vi "Boiler.vi"() -> ()   [LabVIEW 2023]
uses:
  Controls/Boiler Controls.ctl
  Controls/Boiler Simulation Controls.ctl
  Controls/Boiler Status Indicators.ctl
  Controls/State.ctl
  Controls/DataCluster.ctl
panel:
  out "error out":errorcluster
  in  "error in (no error)":errorcluster
  in  "stop":bool
  out "Boiler Status Indicators":T1={"Status"="Lockout", "Primary Fan"=FALSE, "Natural Gas Valve"=FALSE, "Pilot"=FALSE, "Fuel Valve"=FALSE, "Forced Draft Fan"=FALSE, "Time Count"=0.0} {"Time Count" format="%.2g"}
  in  "Boiler Simulation Controls":T2 {"Flame Sensor Value (%)" min=0.0 max=100.0 scale=0.0..100.0}
  in  "Boiler Controls":T3 {"Fuel Valve Position" min=0.0 max=100.0 scale=0.0..100.0 scale format="%.2f"}
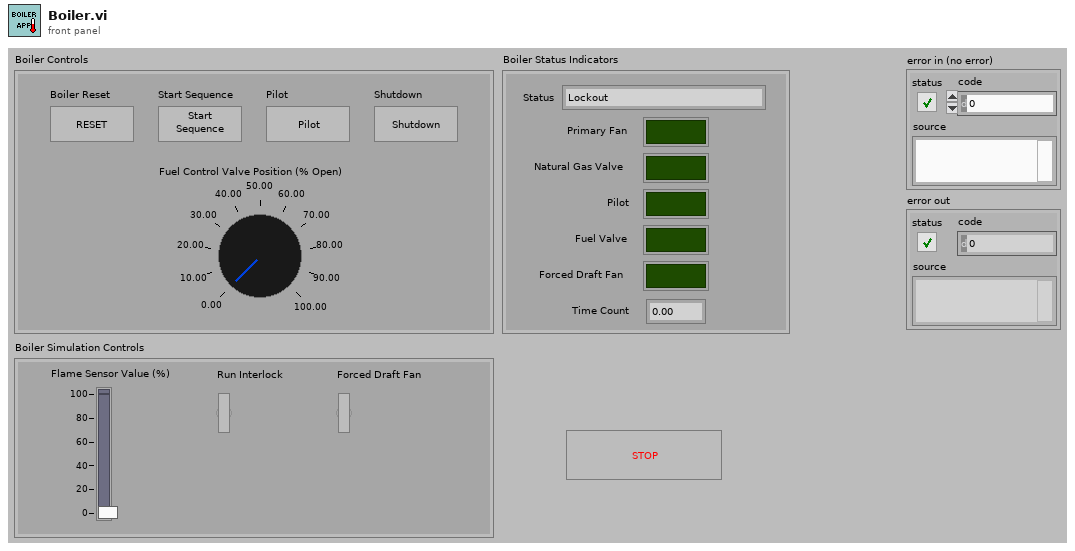
[diagram p1: front panel]
types:
  T1 = typedef "Boiler Status Indicators.ctl" = cluster{"Status":string, "Primary Fan":bool, "Natural Gas Valve":bool, "Pilot":bool, "Fuel Valve":bool, "Forced Draft Fan":bool, "Time Count":dbl}
  T2 = typedef "Boiler Simulation Controls.ctl" = cluster{"Flame Sensor Value (%)":dbl, "Run Interlock":bool, "Forced Draft Fan":bool}
  T3 = typedef "Boiler Controls.ctl" = cluster{"Boiler Reset":bool, "Start Sequence":bool, "Pilot":bool, "Shutdown":bool, "Fuel Valve Position":dbl}
  T4 = typedef "DataCluster.ctl" = cluster{"Boiler Log Path":path, "Last State":T5, "Time out":i32, "Ini Values":cluster{"Timer Count":dbl, "Flame Range Value":dbl, "Valve Position ":cluster{"Min":dbl, "Max":dbl}}, "Flame Sensor Val":dbl, "Fuel Valve Position":dbl, "Timeout Rate":i32}
  T5 = typedef "State.ctl" = enum16{"Boiler Initialized", "Boiler Ready", "Start Pre-Purge", "Pre-Purge Complete", "Pilot On", "Pilot Proved", "Force Draft Fan ON", "Boiler Running", "Start Shutdown Purge", "Shutdown Purge Complete", "Wait for Something"}
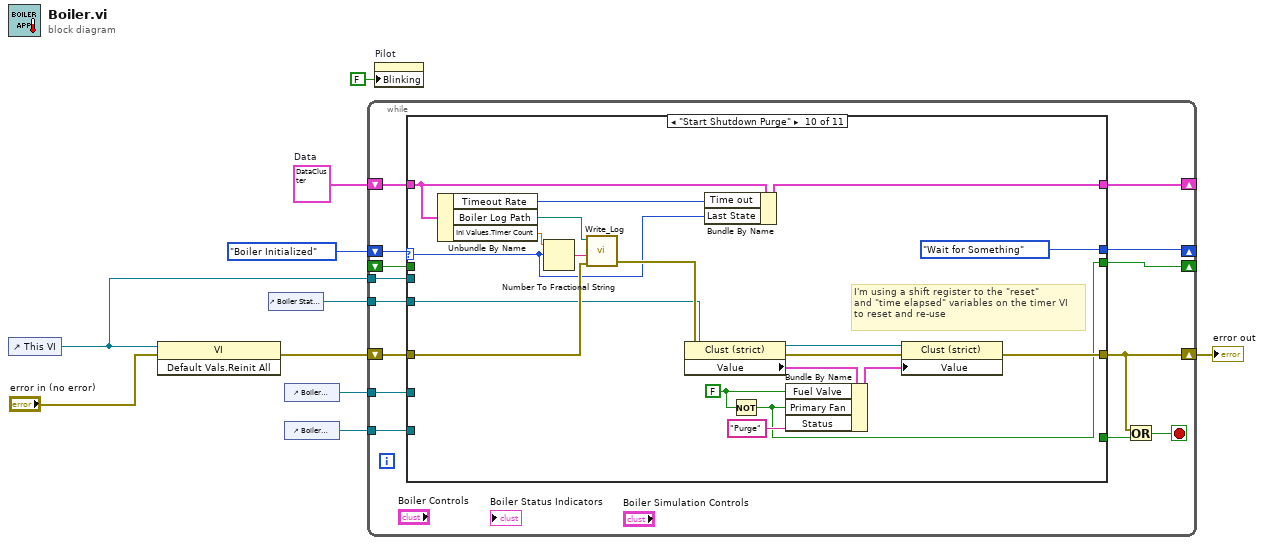
[diagram p0: block diagram]
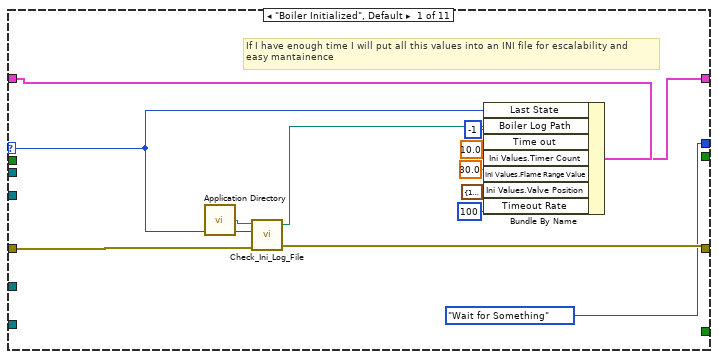
[diagram p2: hidden frame]
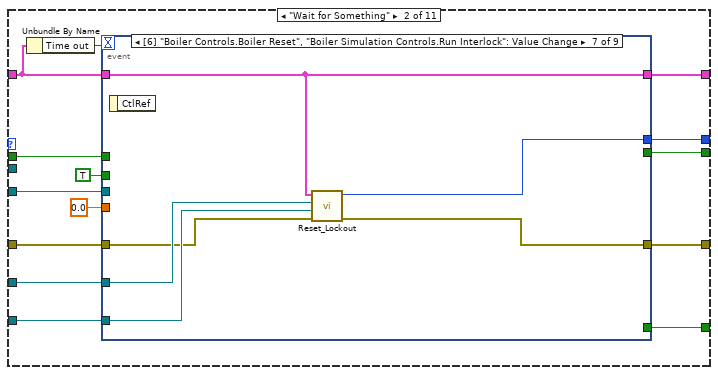
[diagram p3: hidden frame]
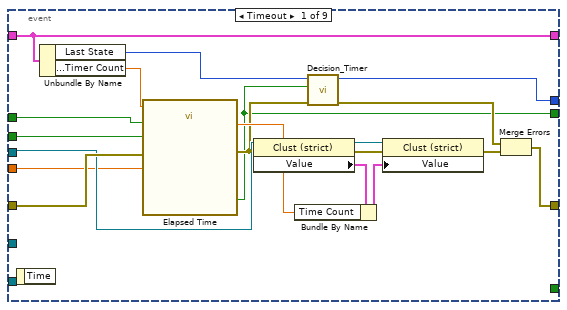
[diagram p4: hidden frame]
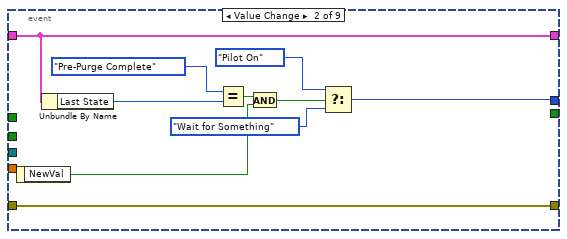
[diagram p5: hidden frame]
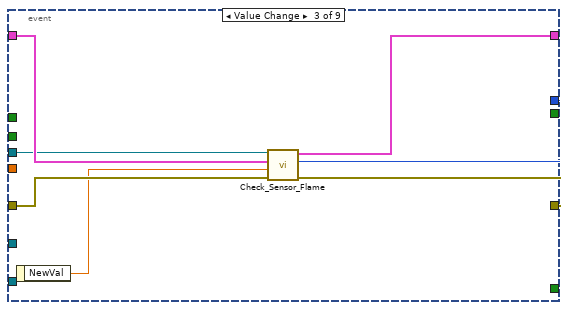
[diagram p6: hidden frame]
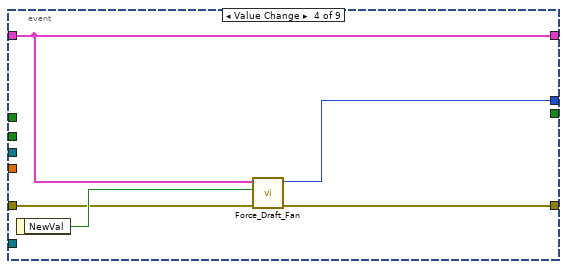
[diagram p7: hidden frame]
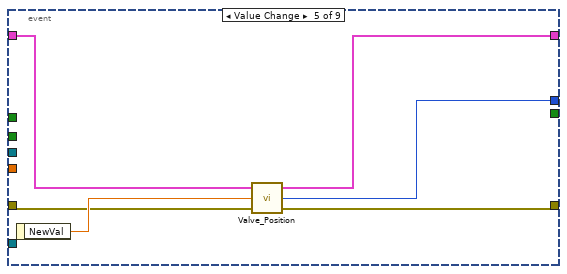
[diagram p8: hidden frame]
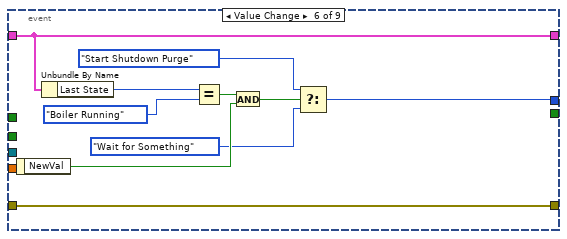
[diagram p9: hidden frame]
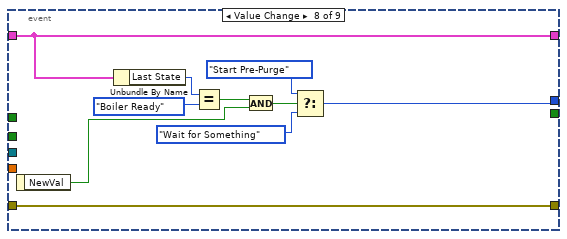
[diagram p10: hidden frame]
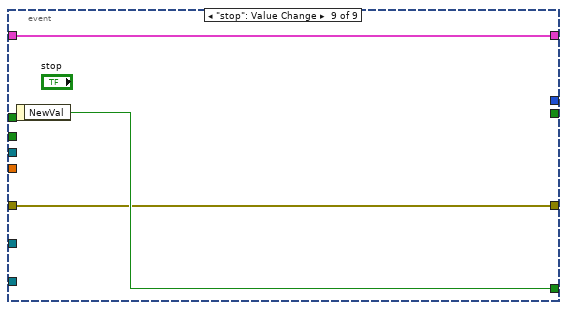
[diagram p11: hidden frame]
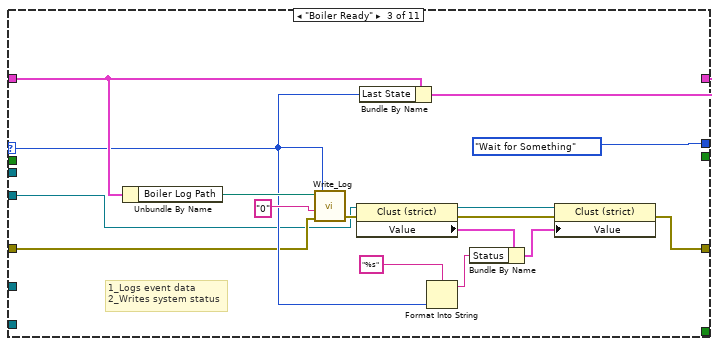
[diagram p12: hidden frame]
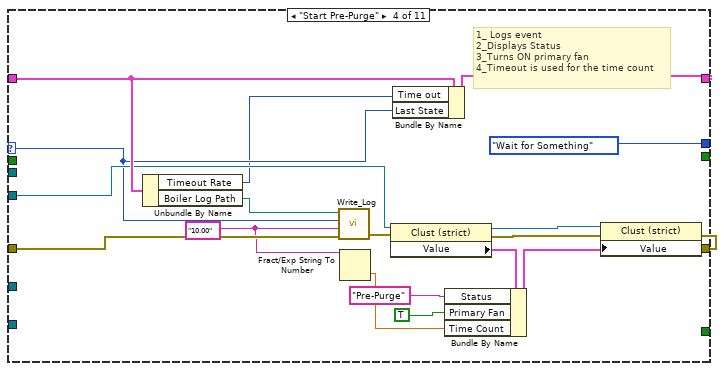
[diagram p13: hidden frame]
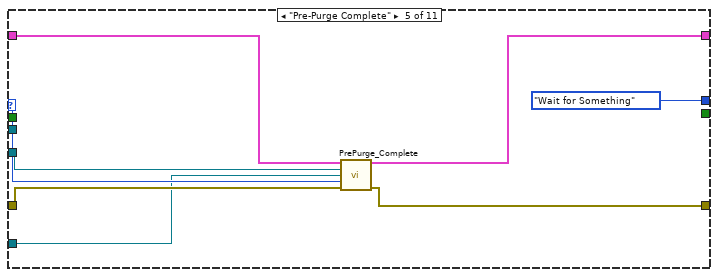
[diagram p14: hidden frame]
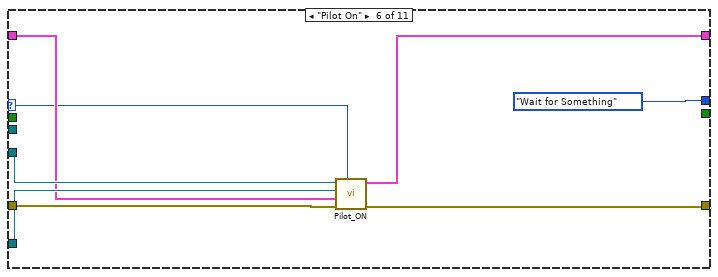
[diagram p15: hidden frame]
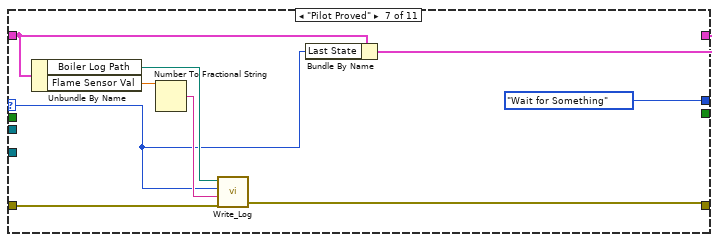
[diagram p16: hidden frame]
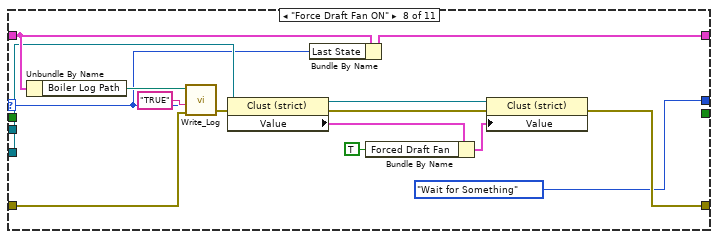
[diagram p17: hidden frame]
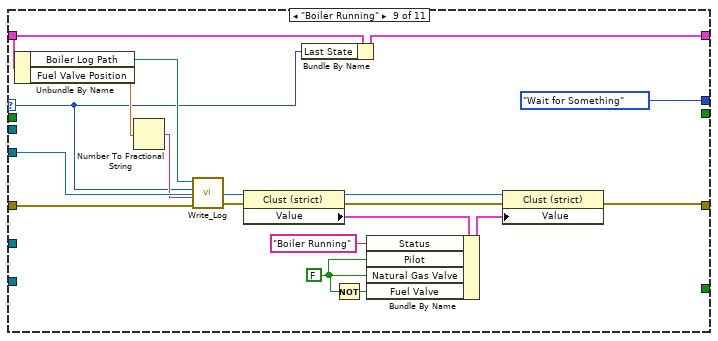
[diagram p18: hidden frame]
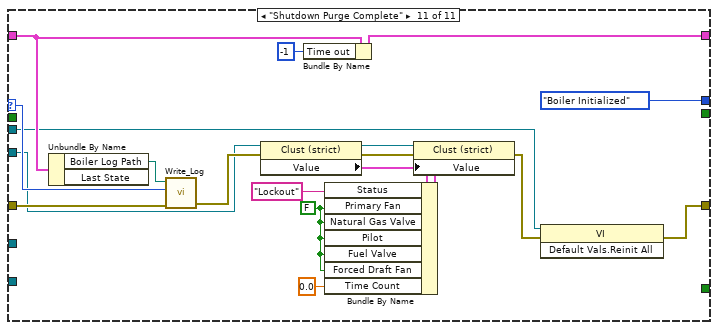
[diagram p19: hidden frame]
diagram:
  w6 = T4 {"Boiler Log Path"=path "", "Last State"=enum."Boiler Initialized", "Time out"=0, "Ini Values"={"Timer Count"=0.0, "Flame Range Value"=0.0, "Valve Position "={"Min"=0.0, "Max"=0.0}}, "Flame Sensor Val"=0.0, "Fuel Valve Position"=0.0, "Timeout Rate"=0}  # Data
  n1 = control-ref of="This VI"() -> (w1:refnum<vi>)
  n2 = invoke class="VI" method="Default Vals.Reinit All"(reference=w1, error in="error in (no error)") -> (error out=w10:errorcluster)  [unwired: 1 in, 2 out]
  n3 = control-ref of="Boiler Status Indicators"() -> (w3:refnum<vi>)
  n4 = control-ref of="Boiler Controls"() -> (w5:refnum<vi>)
  n5 = control-ref of="Boiler Simulation Controls"() -> (w4:refnum<vi>)
  n6 = while {
    shift-right: [w23] -> w8
    shift-left: w10 -> [w24]
    shift-right: [w18] -> _
    shift-left: w6 -> [w19]
    shift-right: [w17] -> _
    shift-left: State."Boiler Initialized" -> [w20]
    tunnel: w5 -> [w16]
    tunnel: w4 -> [w15]
    tunnel: w3 -> [w14]
    shift-right: [w13] -> _
    shift-left: _ -> [w12]
    tunnel: w1 -> [w11]
    stop <- w22 stop-if-true
    n7 = case shown="\"Start Shutdown Purge\"" w20 {
      selector: w20 -> [w31 _ w133 w145 w164 w170 w178 w188 w202 w222 w250]
      tunnel: w24 -> [w36 w51 w132 w157 w168 w174 w186 w201 w209 w235 w254]
      tunnel: [w35 w50 w129 w148 w166 w172 w185 w194 w216 w228 w240] -> w23
      tunnel: [_ w49 _ _ _ _ _ _ _ _ _] -> w21
      tunnel: w19 -> [w37 w43 w140 w161 w169 w173 w184 w199 w207 w237 w252]
      tunnel: [w32 w44 w143 w146 w165 w171 w179 w189 w203 w231 w256] -> w18
      tunnel: [State."Wait for Something" w45 State."Wait for Something" ("State Out") State."Wait for Something" ("State Out") State."Wait for Something" ("State Out") State."Wait for Something" ("State Out") State."Wait for Something" ("State Out") State."Wait for Something" ("State Out") State."Wait for Something" ("State Out") State."Wait for Something" ("State Out") State."Boiler Initialized" ("State Out")] -> w17
      tunnel: w16 -> [_ w48 _ _ w163 w176 _ _ _ _ _]
      tunnel: w15 -> [_ w47 _ _ _ _ _ _ _ _ _]
      tunnel: w14 -> [_ w46 w128 w159 w167 w175 _ w195 w217 w229 w248]
      tunnel: [_ w39 _ _ _ _ _ _ _ w221 _] -> w13
      tunnel: w12 -> [_ w38 _ _ _ _ _ _ _ _ _]
      tunnel: w11 -> [_ _ _ _ _ _ _ _ _ _ w239]
      frame "Boiler Initialized", Default {
        # "If I have enough time I will put all this values into an INI file for escalability and\neasy mantainence"
        n8 = call <vilib>:"Application Directory.vi"() -> ("Application Directory"=w34:path)
        n9 = call "Check_Ini_Log_File.vi"("Application path"=w34, "State"=w31, "error in (no error)"=w36) -> ("Application path"=w30:path, "error out"=w35:errorcluster)  [unwired: 3 in]
        n10 = Bundle By Name(cluster=w37, "Last State"=w31, "Boiler Log Path"=w30, "Time out"=-1, "Ini Values.Timer Count"=10.0 ("Timer Count"), "Ini Values.Flame Range Value"=30.0 ("Ini Values.Flame Value"), "Ini Values.Valve Position"=cluster{"Min":dbl, "Max":dbl} {"Min"=10.0, "Max"=75.0}, "Timeout Rate"=100) -> (w32:T4)
      }
      frame "Wait for Something" {
        n11 = Unbundle By Name(w43) -> ("Time out"=w42:i32)
        n12 = event shown="[6] \"Boiler Controls.Boiler Reset\", \"Boiler Simulation Controls.Run Interlock\": Value Change" {
          selector: _ -> [_ _ _ _ _ _ _ _ _]
          dyn-events: _ -> [_ _ _ _ _ _ _ _ _]
          timeout: w42 -> [_ _ _ _ _ _ _ _ _]
          tunnel: w51 -> [w70 w80 w87 w88 w93 w108 w112 w124 w126]
          tunnel: [w57 w80 w84 w89 w94 w108 w111 w124 w126] -> w50
          tunnel: [_ _ _ _ _ _ _ _ w127] -> w49
          tunnel: w48 -> [_ _ _ _ _ _ w114 _ _]
          tunnel: w47 -> [_ _ _ _ _ _ w113 _ _]
          tunnel: w46 -> [w67 _ w85 _ _ _ _ _ _]
          tunnel: [w60 w73 w83 w91 w97 w101 w110 w117 _] -> w45
          tunnel: w43 -> [w69 w79 w86 w92 w98 w107 w109 w122 w125]
          tunnel: [w69 w79 w82 w92 w96 w107 w109 w122 w125] -> w44
          tunnel: 0.0 ("Set Start Time (s)") -> [w55 _ _ _ _ _ _ _ _]
          tunnel: TRUE ("Auto Reset") -> [w54 _ _ _ _ _ _ _ _]
          tunnel: [w53 _ _ _ _ _ _ _ _] -> w39
          tunnel: w38 -> [w52 _ _ _ _ _ _ _ _]
          event Timeout {
            n13 = event-data() -> ()  [unwired: 1 in, 1 out]
            n14 = Unbundle By Name(w69) -> ("Last State"=w59:T5, "Ini Values.Timer Count"=w68:dbl)
            n15 = call "Elapsed Time"("Time Target (s)"=w68, "Reset"=w52, "Auto Reset"=w54, "error in (no error)"=w70, "Set Start Time (s)"=w55) -> ("Elapsed Time (s)"=w61:dbl, "Time has Elapsed"=w53:bool, "error out"=w58:errorcluster)  [unwired: 7 in, 5 out]
            n16 = property class="Clust (strict)"(reference=w67, error in=w58) -> (reference out=w66:refnum<vi>, error out=w65:errorcluster, "Value"=w63:T1)
            n17 = Bundle By Name(cluster=w63, "Time Count"=w61) -> (w62:T1)
            n18 = call "Decision_Timer.vi"("error in"=w58, "Time has Elapsed"=w53, "Last State"=w59) -> ("error out"=w56:errorcluster, "State"=w60:T5)  [unwired: 7 in]
            n19 = property class="Clust (strict)"(reference=w66, error in=w65, "Value"=w62) -> (error out=w64:errorcluster)  [unwired: 1 out]
            n20 = Merge Errors(w56, w64) -> (w57:errorcluster)
          }
          event Value Change {
            n21 = event-data() -> ("NewVal"=w75:bool)  [unwired: 1 in]
            n22 = Unbundle By Name(w79) -> ("Last State"=w78:T5)
            n23 = Equal?(x=State."Pre-Purge Complete", y=w78) -> (x = y?=w76:bool)
            n24 = And(x=w76, y=w75) -> (x .and. y?=w74:bool)
            n25 = Select(t=State."Pilot On" ("x"), s=w74, f=State."Wait for Something" ("x")) -> (s? t:f=w73:T5)
          }
          event Value Change {
            n26 = event-data() -> ("NewVal"=w81:dbl)  [unwired: 1 in]
            n27 = call "Check_Sensor_Flame.vi"("error in (no error)"=w87, "NewVal"=w81, "Data in"=w86, "Cluster in"=w85) -> ("error out"=w84:errorcluster, "State"=w83:T5, "Data out"=w82:T4)  [unwired: 5 in]
          }
          event Value Change {
            n28 = event-data() -> ("NewVal"=w90:bool)  [unwired: 1 in]
            n29 = call "Force_Draft_Fan.vi"("error in"=w88, "NewVal"=w90, "Data"=w92) -> ("error out"=w89:errorcluster, "State"=w91:T5)  [unwired: 7 in]
          }
          event Value Change {
            n30 = event-data() -> ("NewVal"=w95:dbl)  [unwired: 1 in]
            n31 = call "Valve_Position.vi"("Data in"=w98, "NewVal"=w95, "error in"=w93) -> ("Data out"=w96:T4, "State"=w97:T5, "error out"=w94:errorcluster)  [unwired: 2 in]
          }
          event Value Change {
            n32 = event-data() -> ("NewVal"=w103:bool)  [unwired: 1 in]
            n33 = Unbundle By Name(w107) -> ("Last State"=w106:T5)
            n34 = Equal?(x=w106, y=State."Boiler Running") -> (x = y?=w104:bool)
            n35 = And(x=w104, y=w103) -> (x .and. y?=w102:bool)
            n36 = Select(t=State."Start Shutdown Purge" ("y"), s=w102, f=State."Wait for Something" ("y")) -> (s? t:f=w101:T5)
          }
          event Value Change {
            n37 = event-data() -> ()  [unwired: 1 in, 1 out]
            n38 = call "Reset_Lockout.vi"("error in (no error)"=w112, "Boiler Simulation Controls"=w113, "Boiler Controls"=w114, "Data"=w109) -> ("error out"=w111:errorcluster, "State Out"=w110:T5)  [unwired: 2 in]
          }
          event Value Change {
            n39 = event-data() -> ("NewVal"=w123:bool)  [unwired: 1 in]
            n40 = Unbundle By Name(w122) -> ("Last State"=w121:T5)
            n41 = Equal?(x=w121, y=State."Boiler Ready") -> (x = y?=w119:bool)
            n42 = And(x=w119, y=w123) -> (x .and. y?=w118:bool)
            n43 = Select(t=State."Start Pre-Purge", s=w118, f=State."Wait for Something") -> (s? t:f=w117:T5)
          }
          event "stop": Value Change {
            n44 = event-data() -> ("NewVal"=w127:bool)  [unwired: 1 in]
          }
        }
      }
      frame "Boiler Ready" {
        # "1_Logs event data\n2_Writes system status"
        n45 = Unbundle By Name(w140) -> ("Boiler Log Path"=w139:path)
        n46 = call "Write_Log.vi"("error in (no error)"=w132, "Event data string"="0", "State"=w133, "dup path"=w139) -> ("error out"=w131:errorcluster)  [unwired: 2 in]
        n47 = property class="Clust (strict)"(reference=w128, error in=w131) -> (reference out=w136:refnum<vi>, error out=w130:errorcluster, "Value"=w135:T1)
        n48 = Bundle By Name(cluster=w140, "Last State"=w133) -> (w143:T4)
        n49 = Format Into String(format string="%s", w133) -> (resulting string=w138:string)  [unwired: 2 in, 1 out]
        n50 = Bundle By Name(cluster=w135, "Status"=w138) -> (w134:T1)
        n51 = property class="Clust (strict)"(reference=w136, error in=w130, "Value"=w134) -> (error out=w129:errorcluster)  [unwired: 1 out]
      }
      frame "Start Pre-Purge" {
        w151 = "10.00"
        # "1_ Logs event\n2_Displays Status\n3_Turns ON primary fan\n4_Timeout is used for the time count"
        n52 = Unbundle By Name(w161) -> ("Timeout Rate"=w144:i32, "Boiler Log Path"=w160:path)
        n53 = call "Write_Log.vi"("error in (no error)"=w157, "Event data string"=w151, "State"=w145, "dup path"=w160) -> ("error out"=w149:errorcluster)  [unwired: 2 in]
        n54 = Fract/Exp String To Number(string=w151) -> (number=w150:dbl)  [unwired: 3 in, 1 out]
        n55 = property class="Clust (strict)"(reference=w159, error in=w149) -> (reference out=w158:refnum<vi>, error out=w156:errorcluster, "Value"=w155:T1)
        n56 = Bundle By Name(cluster=w161, "Time out"=w144, "Last State"=w145) -> (w146:T4)
        n57 = Bundle By Name(cluster=w155, "Status"="Pre-Purge", "Primary Fan"=TRUE, "Time Count"=w150) -> (w154:T1)
        n58 = property class="Clust (strict)"(reference=w158, error in=w156, "Value"=w154) -> (error out=w148:errorcluster)  [unwired: 1 out]
      }
      frame "Pre-Purge Complete" {
        n59 = call "PrePurge_Complete.vi"("Data in"=w169, "Boiler Status Indicators"=w167, "Boiler Controls"=w163, "State"=w164, "error in (no error)"=w168) -> ("Data out"=w165:T4, "error out"=w166:errorcluster)  [unwired: 9 in]
      }
      frame "Pilot On" {
        n60 = call "Pilot_ON.vi"("State"=w170, "error in (no error)"=w174, "Data in"=w173, 10:"Boiler Controls"=w176, 11:"Boiler Controls"=w175) -> ("error out"=w172:errorcluster, "Data out"=w171:T4)  [unwired: 5 in]
      }
      frame "Pilot Proved" {
        n61 = Unbundle By Name(w184) -> ("Boiler Log Path"=w183:path, "Flame Sensor Val"=w182:dbl)
        n62 = Number To Fractional String(number=w182) -> (F-format string=w181:string)  [unwired: 3 in]
        n63 = call "Write_Log.vi"("error in (no error)"=w186, "Event data string"=w181, "State"=w178, "dup path"=w183) -> ("error out"=w185:errorcluster)  [unwired: 2 in]
        n64 = Bundle By Name(cluster=w184, "Last State"=w178) -> (w179:T4)
      }
      frame "Force Draft Fan ON" {
        n65 = Unbundle By Name(w199) -> ("Boiler Log Path"=w198:path)
        n66 = call "Write_Log.vi"("error in (no error)"=w201, "Event data string"="TRUE", "State"=w188, "dup path"=w198) -> ("error out"=w200:errorcluster)  [unwired: 2 in]
        n67 = property class="Clust (strict)"(reference=w195, error in=w200) -> (reference out=w193:refnum<vi>, error out=w196:errorcluster, "Value"=w192:T1)
        n68 = Bundle By Name(cluster=w199, "Last State"=w188) -> (w189:T4)
        n69 = Bundle By Name(cluster=w192, "Forced Draft Fan"=TRUE) -> (w191:T1)
        n70 = property class="Clust (strict)"(reference=w193, error in=w196, "Value"=w191) -> (error out=w194:errorcluster)  [unwired: 1 out]
      }
      frame "Boiler Running" {
        w210 = FALSE
        n71 = Unbundle By Name(w207) -> ("Boiler Log Path"=w206:path, "Fuel Valve Position"=w205:dbl)
        n72 = Number To Fractional String(number=w205) -> (F-format string=w204:string)  [unwired: 3 in]
        n73 = call "Write_Log.vi"("error in (no error)"=w209, "Event data string"=w204, "State"=w202, "dup path"=w206) -> ("error out"=w208:errorcluster)  [unwired: 2 in]
        n74 = property class="Clust (strict)"(reference=w217, error in=w208) -> (reference out=w215:refnum<vi>, error out=w218:errorcluster, "Value"=w214:T1)
        n75 = Bundle By Name(cluster=w207, "Last State"=w202) -> (w203:T4)
        n76 = Not(x=w210) -> (.not. x?=w211:bool)
        n77 = Bundle By Name(cluster=w214, "Status"="Boiler Running", "Pilot"=w210, "Natural Gas Valve"=w210, "Fuel Valve"=w211) -> (w213:T1)
        n78 = property class="Clust (strict)"(reference=w215, error in=w218, "Value"=w213) -> (error out=w216:errorcluster)  [unwired: 1 out]
      }
      frame "Start Shutdown Purge" {
        w224 = FALSE ("Fuel Valve")
        # "I'm using a shift register to the \"reset\"\nand \"time elapsed\" variables on the timer VI\nto reset and re-use"
        n79 = Unbundle By Name(w237) -> ("Timeout Rate"=w220:i32, "Boiler Log Path"=w236:path, "Ini Values.Timer Count"=w233:dbl)
        n80 = Number To Fractional String(number=w233) -> (F-format string=w232:string)  [unwired: 3 in]
        n81 = call "Write_Log.vi"("error in (no error)"=w235, "Event data string"=w232, "State"=w222, "dup path"=w236) -> ("error out"=w234:errorcluster)  [unwired: 2 in]
        n82 = property class="Clust (strict)"(reference=w229, error in=w234) -> (reference out=w227:refnum<vi>, error out=w230:errorcluster, "Value"=w226:T1)
        n83 = Bundle By Name(cluster=w237, "Time out"=w220, "Last State"=w222) -> (w231:T4)
        n84 = Not(x=w224) -> (.not. x?=w221:bool)
        n85 = Bundle By Name(cluster=w226, "Fuel Valve"=w224, "Primary Fan"=w221, "Status"="Purge") -> (w225:T1)
        n86 = property class="Clust (strict)"(reference=w227, error in=w230, "Value"=w225) -> (error out=w228:errorcluster)  [unwired: 1 out]
      }
      frame "Shutdown Purge Complete" {
        w243 = FALSE ("Primary Fan")
        n87 = Unbundle By Name(w252) -> ("Boiler Log Path"=w251:path)  [unwired: 1 out]
        n88 = call "Write_Log.vi"("error in (no error)"=w254, "State"=w250, "dup path"=w251) -> ("error out"=w253:errorcluster)  [unwired: 3 in]
        n89 = property class="Clust (strict)"(reference=w248, error in=w253) -> (reference out=w247:refnum<vi>, error out=w249:errorcluster, "Value"=w246:T1)
        n90 = Bundle By Name(cluster=w252, "Time out"=-1) -> (w256:T4)
        n91 = Bundle By Name(cluster=w246, "Status"="Lockout", "Primary Fan"=w243, "Natural Gas Valve"=w243, "Pilot"=w243, "Fuel Valve"=w243, "Forced Draft Fan"=w243, "Time Count"=0.0) -> (w245:T1)
        n92 = property class="Clust (strict)"(reference=w247, error in=w249, "Value"=w245) -> (error out=w241:errorcluster)  [unwired: 1 out]
        n93 = invoke class="VI" method="Default Vals.Reinit All"(reference=w239, error in=w241) -> (error out=w240:errorcluster)  [unwired: 1 in, 2 out]
      }
    }
    n94 = Or(x=w23, y=w21) -> (x .or. y?=w22:bool)
  }
  "error out" <- w8
  n95 = property on="Pilot" class="Bool (strict)"("Blinking"=FALSE) -> ()  [unwired: 2 in, 2 out]
